vi "RefChVout.vi"(0 "Vout  P 4":refnum<vi>, 1 "Vout  P 5":refnum<vi>, 2 "Vout  P 6":refnum<vi>, 3 "Init_F":bool=TRUE, 4 "Vout  P 7":refnum<vi>, 5 "Vout  P 8":refnum<vi>, 6 "Vout  P 9":refnum<vi>, 8 "Vout  P 3":refnum<vi>, 9 "Vout  P 10":refnum<vi>, 10 "Vout  P 2":refnum<vi>, 11 "Vout  P 11":refnum<vi>, 12 "Vout  P 1":refnum<vi>, 13 "Vout  P 12":refnum<vi>, 27 "error in":errorcluster) -> (7 "error out":errorcluster, 15 "Vout  P1 out":refnum<vi>, 16 "Vout  P12 out":refnum<vi>, 17 "Vout  P2 out":refnum<vi>, 18 "Vout  P11 out":refnum<vi>, 19 "Vout  P3 out":refnum<vi>, 20 "Vout  P10 out":refnum<vi>, 21 "Vout  P9 out":refnum<vi>, 22 "Vout  P8 out":refnum<vi>, 23 "Vout  P7 out":refnum<vi>, 24 "Vout  P6 out":refnum<vi>, 25 "Vout  P5 out":refnum<vi>, 26 "Vout  P4 out":refnum<vi>)   [LabVIEW 2017]
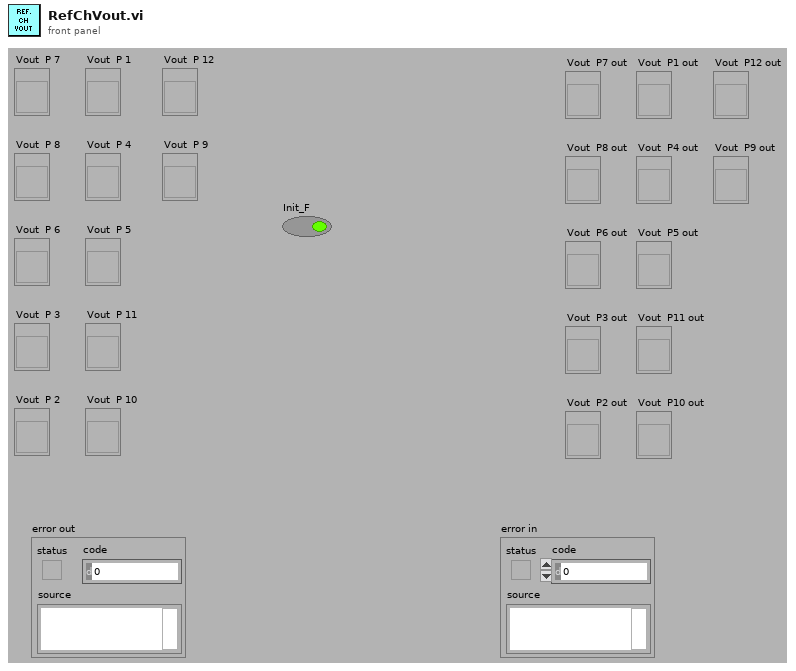
[diagram p1: front panel]
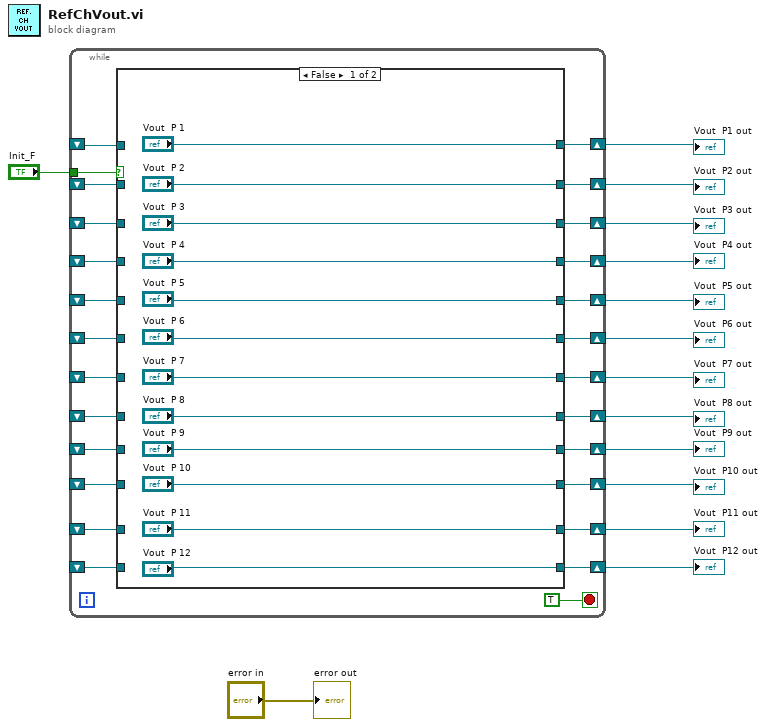
[diagram p0: block diagram]
diagram:
  n1 = while {
    shift-right: [w39] -> w12
    shift-left: _ -> [w38]
    tunnel: "Init_F" -> [w37]
    shift-right: [w36] -> w11
    shift-left: _ -> [w29]
    shift-right: [w35] -> w10
    shift-left: _ -> [w28]
    shift-right: [w34] -> w9
    shift-left: _ -> [w23]
    shift-right: [w33] -> w8
    shift-left: _ -> [w27]
    shift-right: [w32] -> w7
    shift-left: _ -> [w26]
    shift-right: [w31] -> w6
    shift-left: _ -> [w25]
    shift-right: [w30] -> w5
    shift-left: _ -> [w24]
    shift-right: [w22] -> w4
    shift-left: _ -> [w20]
    shift-right: [w21] -> w3
    shift-left: _ -> [w19]
    shift-right: [w18] -> w2
    shift-left: _ -> [w16]
    shift-right: [w17] -> w1
    shift-left: _ -> [w15]
    stop <- TRUE stop-if-true
    n2 = case shown="False" w37 {
      tunnel: ["Vout  P 1" w64] -> w39
      tunnel: w38 -> [_ w64]
      tunnel: ["Vout  P 2" w57] -> w36
      tunnel: ["Vout  P 3" w58] -> w35
      tunnel: ["Vout  P 4" w59] -> w34
      tunnel: ["Vout  P 5" w60] -> w33
      tunnel: ["Vout  P 6" w61] -> w32
      tunnel: ["Vout  P 7" w62] -> w31
      tunnel: ["Vout  P 8" w63] -> w30
      tunnel: w29 -> [_ w57]
      tunnel: w28 -> [_ w58]
      tunnel: w27 -> [_ w60]
      tunnel: w26 -> [_ w61]
      tunnel: w25 -> [_ w62]
      tunnel: w24 -> [_ w63]
      tunnel: w23 -> [_ w59]
      tunnel: ["Vout  P 9" w56] -> w22
      tunnel: ["Vout  P 10" w55] -> w21
      tunnel: w20 -> [_ w56]
      tunnel: w19 -> [_ w55]
      tunnel: ["Vout  P 11" w54] -> w18
      tunnel: ["Vout  P 12" w53] -> w17
      tunnel: w16 -> [_ w54]
      tunnel: w15 -> [_ w53]
      frame False {
      }
      frame True {
      }
    }
  }
  "Vout  P1 out" <- w12
  "Vout  P2 out" <- w11
  "Vout  P3 out" <- w10
  "Vout  P4 out" <- w9
  "Vout  P5 out" <- w8
  "Vout  P6 out" <- w7
  "Vout  P7 out" <- w6
  "Vout  P8 out" <- w5
  "Vout  P9 out" <- w4
  "Vout  P10 out" <- w3
  "Vout  P11 out" <- w2
  "Vout  P12 out" <- w1
  "error out" <- "error in"
